vi "destoryEvents.vi"(8 "error in (no error)":errorcluster, 11 "SettingsEventsManager in":refnum<class "SettingsEventsManager.lvclass">) -> (0 "error out":errorcluster, 3 "SettingsEventsManager out":refnum<class "SettingsEventsManager.lvclass">)   [LabVIEW 2011, in "Tools.lvlib" / "Settings.lvlib" / "SettingsEventsManager.lvclass"]
uses:
  SettingsEventsManager.lvclass
  SettingsEventsManager.lvclass/SettingsEventsManager.ctl
  Settings.lvlib
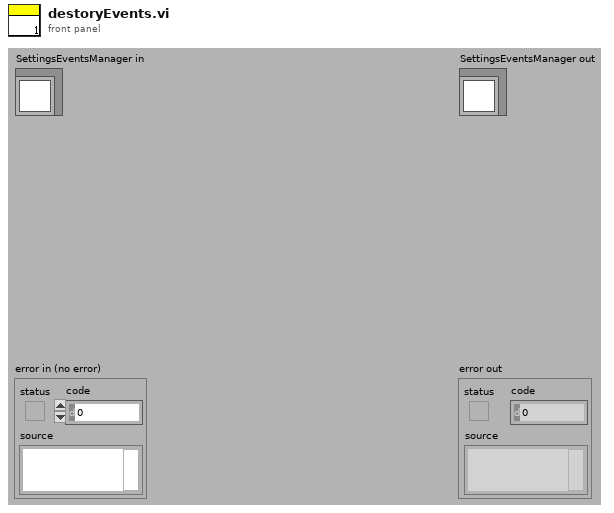
[diagram p1: front panel]
types:
  T1 = cluster{"settingsFrontEndEvents":cluster{"loadSettingsFromPath":refnum<user-event>, "lookUpElementEvent":refnum<user-event>, "saveSettings":refnum<user-event>, "loadSettings":refnum<user-event>, "close":refnum<user-event>, "replaceElement":refnum<user-event>, "findParentNodes":refnum<user-event>, "createNode":refnum<user-event>}, "settingBackEndEvents":cluster{"defaultSettingsPathRequest":refnum<user-event>, "searchResultEvent":refnum<user-event>, "settingsSaved":refnum<user-event>, "settingsLoaded":refnum<user-event>, "foundParentNode":refnum<user-event>}}
  T2 = cluster{"loadSettingsFromPath":refnum<user-event>, "lookUpElementEvent":refnum<user-event>, "saveSettings":refnum<user-event>, "loadSettings":refnum<user-event>, "close":refnum<user-event>, "replaceElement":refnum<user-event>, "findParentNodes":refnum<user-event>, "createNode":refnum<user-event>}
  T3 = cluster{"defaultSettingsPathRequest":refnum<user-event>, "searchResultEvent":refnum<user-event>, "settingsSaved":refnum<user-event>, "settingsLoaded":refnum<user-event>, "foundParentNode":refnum<user-event>}
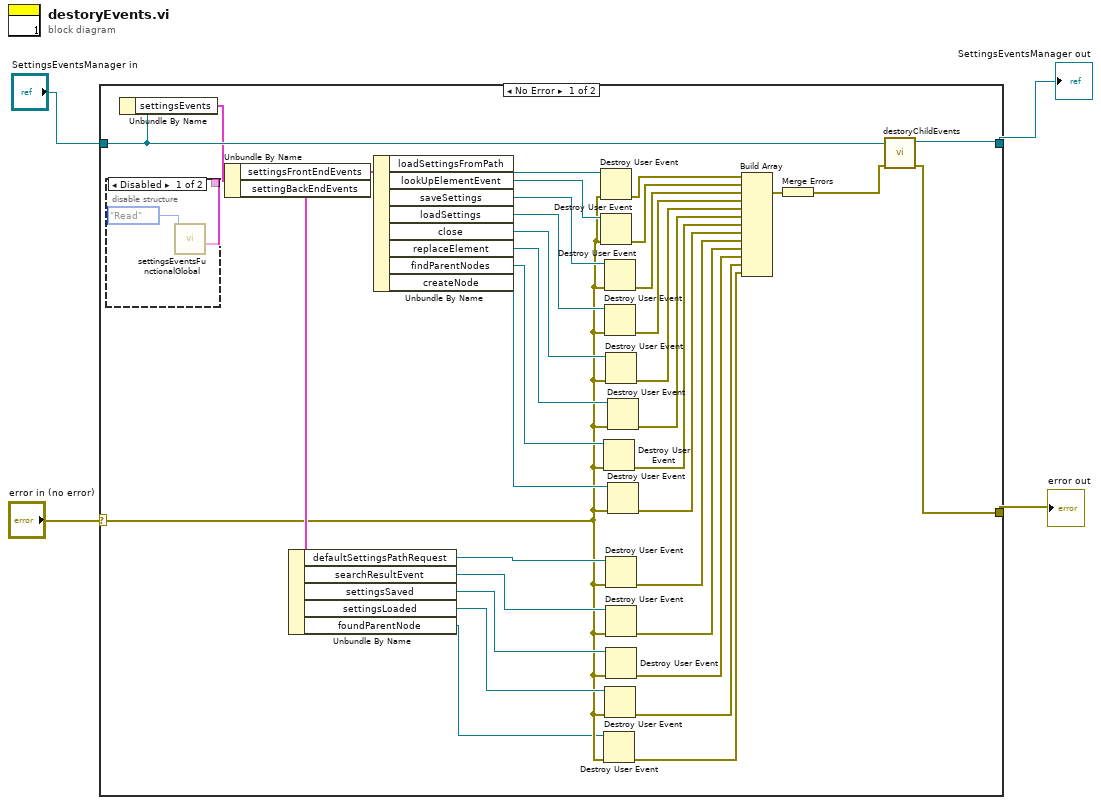
[diagram p0: block diagram]
diagram:
  n1 = case shown="No Error" "error in (no error)" {
    selector: "error in (no error)" -> [w11 w43]
    tunnel: [w18 w43] -> w3
    tunnel: [w20 w42] -> w1
    tunnel: "SettingsEventsManager in" -> [w6 w42]
    frame No Error {
      n2 = disable-structure shown="Disabled" {
        disable-tunnel: [w40 _] -> _
        frame Disabled {
          n3 = call "settingsEventsFunctionalGlobal.vi"("Action"=enum16{"Write", "Read"}."Read") -> ("settingsEvents"=w40:T1)  [unwired: 10 in]
        }
        frame Enabled {
        }
      }
      n4 = Unbundle By Name(w6) -> ("settingsEvents"=w5:T1)
      n5 = Unbundle By Name(w5) -> ("settingsFrontEndEvents"=w39:T2, "settingBackEndEvents"=w34:T3)
      n6 = Unbundle By Name(w34) -> ("defaultSettingsPathRequest"=w30:refnum<user-event>, "searchResultEvent"=w31:refnum<user-event>, "settingsSaved"=w32:refnum<user-event>, "settingsLoaded"=w33:refnum<user-event>, "foundParentNode"=w10:refnum<user-event>)
      n7 = Unbundle By Name(w39) -> ("loadSettingsFromPath"=w38:refnum<user-event>, "lookUpElementEvent"=w37:refnum<user-event>, "saveSettings"=w36:refnum<user-event>, "loadSettings"=w35:refnum<user-event>, "close"=w17:refnum<user-event>, "replaceElement"=w15:refnum<user-event>, "findParentNodes"=w13:refnum<user-event>, "createNode"=w12:refnum<user-event>)
      n8 = Destroy User Event(user event=w38, error in=w11) -> (error out=w29:errorcluster)
      n9 = Destroy User Event(user event=w37, error in=w11) -> (error out=w28:errorcluster)
      n10 = Destroy User Event(user event=w13, error in=w11) -> (error out=w9:errorcluster)
      n11 = Destroy User Event(user event=w10, error in=w11) -> (error out=w7:errorcluster)
      n12 = Destroy User Event(user event=w36, error in=w11) -> (error out=w27:errorcluster)
      n13 = Destroy User Event(user event=w35, error in=w11) -> (error out=w26:errorcluster)
      n14 = Destroy User Event(user event=w33, error in=w11) -> (error out=w22:errorcluster)
      n15 = Destroy User Event(user event=w17, error in=w11) -> (error out=w16:errorcluster)
      n16 = Destroy User Event(user event=w30, error in=w11) -> (error out=w25:errorcluster)
      n17 = Destroy User Event(user event=w31, error in=w11) -> (error out=w24:errorcluster)
      n18 = Destroy User Event(user event=w32, error in=w11) -> (error out=w23:errorcluster)
      n19 = Destroy User Event(user event=w15, error in=w11) -> (error out=w14:errorcluster)
      n20 = Destroy User Event(user event=w12, error in=w11) -> (error out=w8:errorcluster)
      n21 = Build Array(w29, w28, w27, w26, w16, w14, w9, w8, w25, w24, w23, w22, w7) -> (w21:errorcluster[])
      n22 = Merge Errors(w21) -> (w19:errorcluster)
      n23 = call-dynamic "destoryChildEvents.vi"("error in (no error)"=w19, "SettingsEventsManager in"=w6) -> ("error out"=w18:errorcluster, "SettingsEventsManager out"=w20:refnum<class "SettingsEventsManager.lvclass">)  [unwired: 8 in]
    }
    frame Error {
    }
  }
  "error out" <- w3
  "SettingsEventsManager out" <- w1
